vi "Trans-FPGA.vi"() -> ()   [LabVIEW 2016]
uses:
  <vilib>/LabVIEW Targets/FPGA/cRIO/shared/nicrio_ModuleControls/nicrio_cRIO-9871_BaudRateEnum.ctl
  <vilib>/LabVIEW Targets/FPGA/cRIO/shared/nicrio_ModuleControls/nicrio_cRIO-9871_DataBitsEnum.ctl
  <vilib>/LabVIEW Targets/FPGA/cRIO/shared/nicrio_ModuleControls/nicrio_cRIO-9871_ParityEnum.ctl
  <vilib>/LabVIEW Targets/FPGA/cRIO/shared/nicrio_ModuleControls/nicrio_cRIO-9871_StopBitsEnum.ctl
  <vilib>/Platform/TimedLoop/XDataNode/timing_clust.ctl
  <vilib>/Platform/TimedLoop/XDataNode/nitl_modes.ctl
  <vilib>/Platform/TimedLoop/XDataNode/wakeup.ctl
  <vilib>/rvi/FXPMathLib/basic elements/FxpIntAccumulator/subVIs/nifxpmath_IntAccumulator_SimConfig.ctl
  <vilib>/rvi/Emulation/niFpgaGetClockAttributes.vi
  <vilib>/rvi/Emulation/niFpgaSctlEmulationGetInTimedLoop.vi
  <vilib>/rvi/Emulation/niFpgaEmulationReportErrorSimple.vi
  <vilib>/rvi/eio/common/nirviEmuTemplateMethod_errors.vi
  <vilib>/rvi/Emulation/niFpgaCriticalErrorInLSC.vi
  <vilib>/rvi/Analysis/common/codeGenErrors/XNode/niFpgaXNodeCodeGenErrorHandle.vi
  <vilib>/rvi/FXPMathLib/basic elements/FxpIntAccumulator/simVIs/DllFxpIntAccumulator_sub.vi
  <vilib>/rvi/eio/common/nirviEmuTemplatePropertySet_noerrors.vi
  <vilib>/eio/EIONode/EIONode.xnode
  <vilib>/eio/EIOMethodNode/EIOMethodNode.xnode
  <vilib>/rvi/Analysis/measure/dc-rms/XNode/niFpgaDC-RMS.xnode
  <vilib>/Platform/TimedLoop/XDataNode/XDataNode.xnode
  <vilib>/rvi/FXPMathLib/basic elements/FxpIntAccumulator/XNode/nifxpmath_IntAccumulator.xnode
  <vilib>/rvi/FXPMathLib/FxpMul/XNode/nifxpmath_Multiplier.xnode
  <vilib>/eio/EIOPropertyNode/EIOPropertyNode.xnode
  <vilib>/Platform/TimedLoop/XDataNode/XDNodeRunTimeDep.lvlib
  <vilib>/rvi/FXPMathLib/sim/FxpSim.dll
  <vilib>/rvi/eio/common/nirviEmuTemplatePropertyGet_errors.vi
  <vilib>/rvi/eio/common/nirviEmuTemplatePropertyGet_noerrors.vi
  <vilib>/rvi/eio/common/nirviEmuTemplatePropertySet_errors.vi
panel:
  in  "RT error":bool
  in  "switch mag ps set":u8[](array[numeric])=[0, 0, 0, 0, 0, 0, 0, 0, 0, 0]
  out "Switch mag data":u8
  out "Timed Out 2":bool
  out "switch mag field":u8[](array[numeric])
  out "error out 2":errorcluster
  in  "trans ExB mag ps set":u8[](array[numeric])=[0, 0, 0, 0, 0, 0, 0, 0, 0, 0]
  in  "analyzer mag ps set":u8[](array[numeric])=[0, 0, 0, 0, 0, 0, 0, 0, 0, 0]
  out "analyzer mag data":u8
  out "Timed Out":bool
  out "analyzer mag field":u8[](array[numeric])
  out "error out":errorcluster
  out "Ion gauge 4":u8[](array[numeric])
  out "Convectron 4":u8[](array[numeric])
  out "Convectron 3":u8[](array[numeric])
  out "Ion gauge 3":u8[](array[numeric])
  out "Ion gauge 2":u8[](array[numeric])
  out "Convectron 2":u8[](array[numeric])
  out "Convectron 1":u8[](array[numeric])
  out "Ion gauge 1":u8[](array[numeric])
  in  "Analog Output":fxp<+/-,26,5>[](array[numeric])=[0.0, 0.0, 0.0, 0.0, 0.0, 0.0, 0.0, 0.0] format="%.23g"
  out "Analog input":fxp<+/-,26,5>[](array[numeric]) format="%.23g"
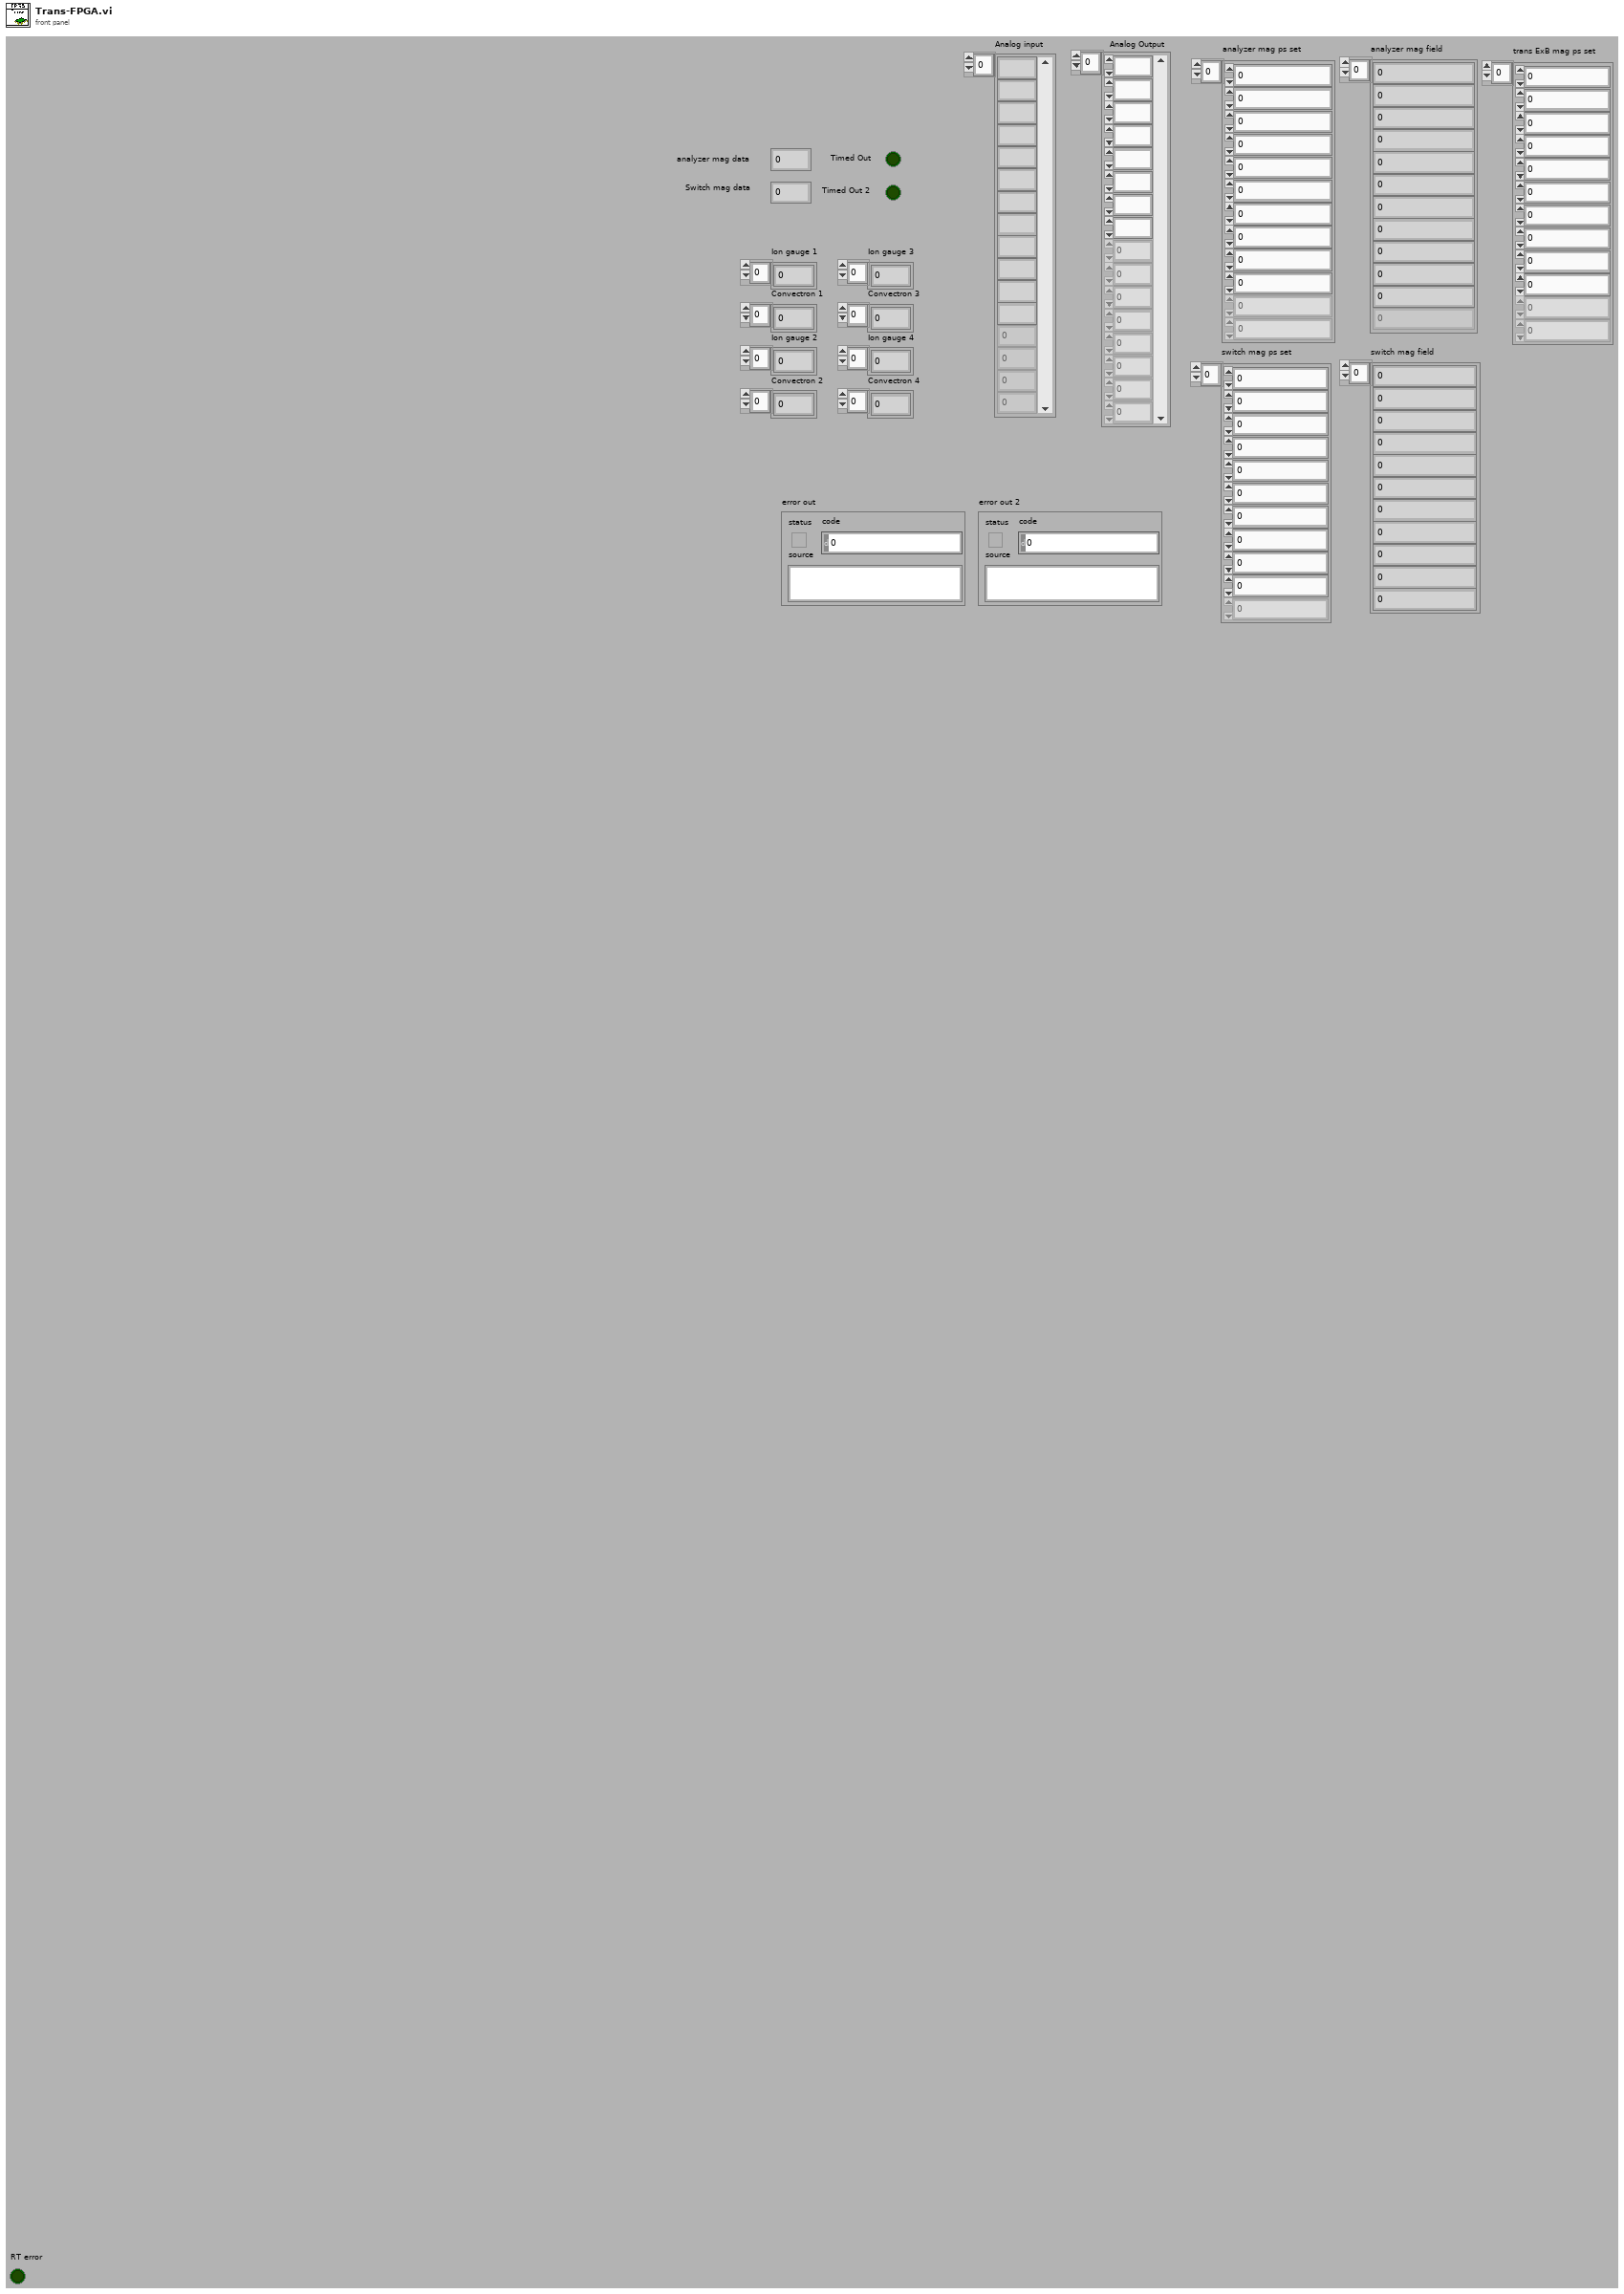
[diagram p1: front panel]
types:
  T1 = typedef "nicrio_cRIO-9871_ParityEnum.ctl" = enum8{"None", "Odd", "Even", "Mark", "Space"}
  T2 = typedef "nicrio_cRIO-9871_StopBitsEnum.ctl" = enum8{"1", "1.5", "2"}
  T3 = typedef "nicrio_cRIO-9871_BaudRateEnum.ctl" = enum16{"75 bps", "110 bps", "134 bps", "150 bps", "300 bps", "600 bps", "1200 bps", "1800 bps", "2400 bps", "4800 bps", "7200 bps", "9600 bps", "14.4 kbps", "19.2 kbps", "28.8 kbps", "38.4 kbps", "57.6 kbps", "115.2 kbps", "230.4 kbps", "460.8 kbps", "921.6 kbps"}
  T4 = typedef "nicrio_cRIO-9871_DataBitsEnum.ctl" = enum8{"5", "6", "7", "8"}
  T5 = typedef "XDNodeRunTimeDep.lvlib/timing_clust.ctl" = cluster{"Expected End [f-1]":u64, "Actual End [f-1]":u64, "Finished Late? [f-1]":bool, "Expected End [i-1]":u64, "Actual End [i-1]":u64, "Finished Late? [i-1]":bool, "Expected Start [i]":u64, "Actual Start [i]":u64, "Expected Start [f]":u64, "Actual Start [f]":u64, "Source Name":string, "Structure Name":string, "Period":i64, "Deadline":i64, "Offset":i64, "Start":i64, "Priority":i32, "Timeout":i32, "Mode":T6, "Wakeup Reason":T7, "Error":errorcluster, "Source Type":string, "Secondary Source Type":string, "Global End Time":u64, "Global Start Time":u64, "Frame Duration":u64, "Iteration Duration":u64, "Assigned CPU":i32, "I/O Scan Engine Mode":u32}
  T6 = typedef "XDNodeRunTimeDep.lvlib/nitl_modes.ctl" = enum32{"No Change", "Process missed periods, maintain original phase", "Discard missed periods, maintain original phase", "Process missed periods, ignore original phase", "Discard missed periods, ignore original phase"}
  T7 = typedef "XDNodeRunTimeDep.lvlib/wakeup.ctl" = enum32{"Normal", "Aborted", "Asynchronous wakeup", "Timing source error", "Timed loop error", "Timeout"}
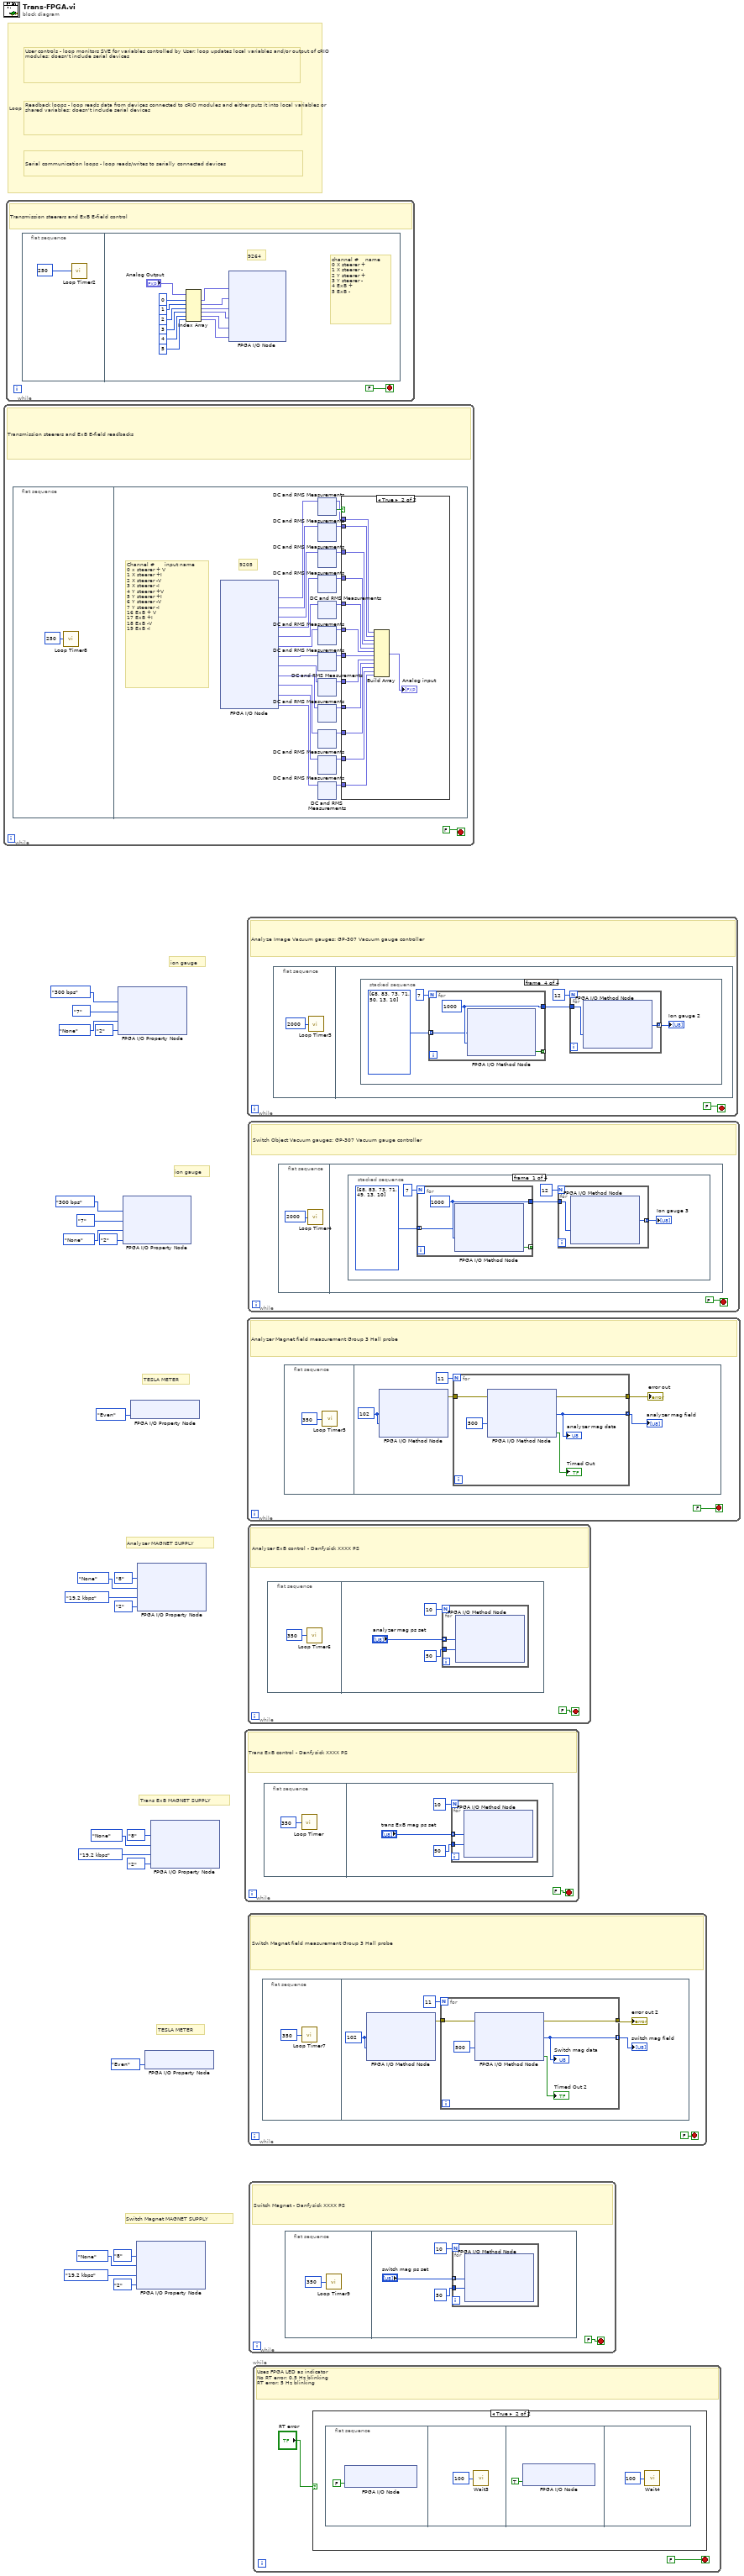
[diagram p0: block diagram]
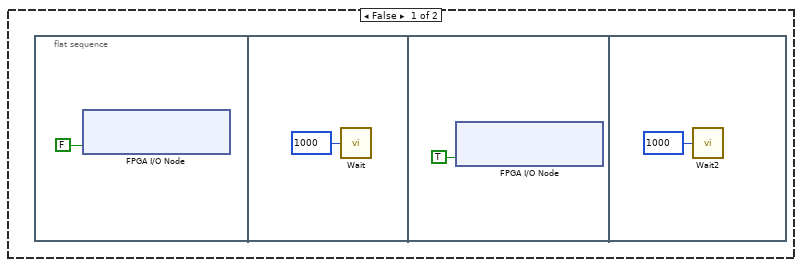
[diagram p2: hidden frame]
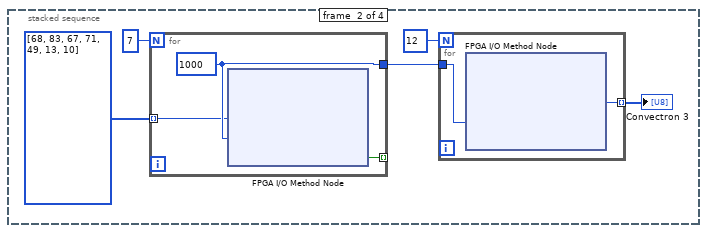
[diagram p4: hidden frame]
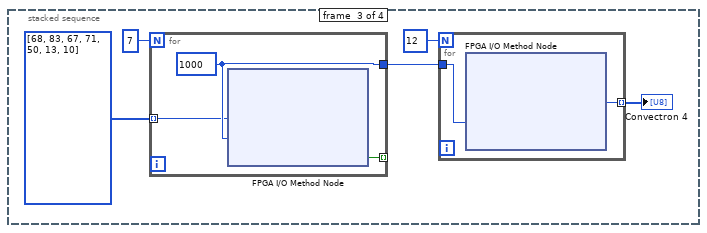
[diagram p5: hidden frame]
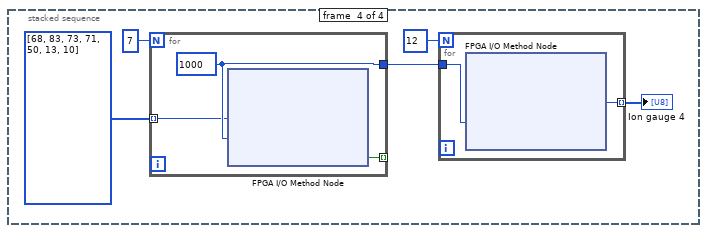
[diagram p6: hidden frame]
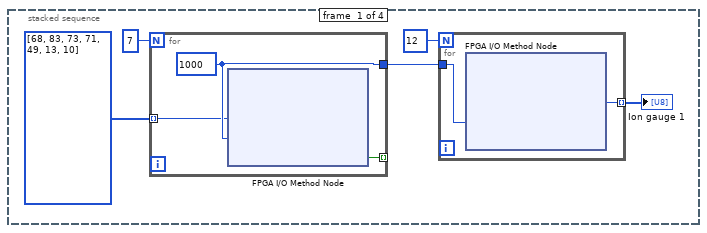
[diagram p7: hidden frame]
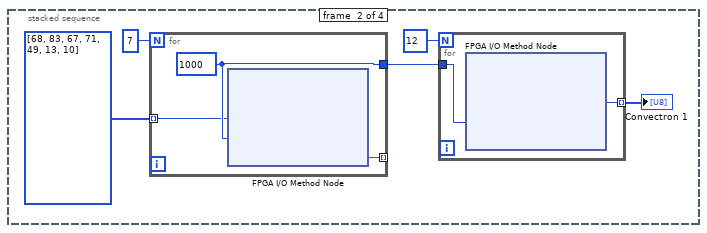
[diagram p8: hidden frame]
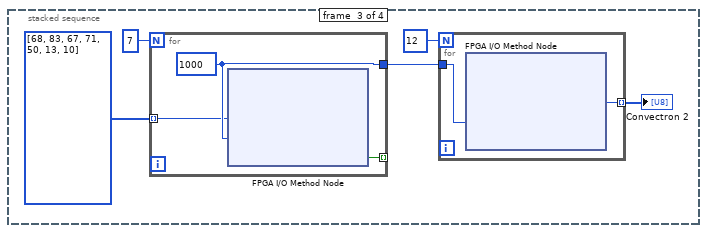
[diagram p9: hidden frame]
diagram:
  # "Serial communication loops - loop reads/writes to serially connected devices"
  # "Readback loops - loop reads data from devices connected to cRIO modules and either puts it into local variables or shared variables; doesn't include serial devices"
  # "User controls - loop monitors SVE for variables controlled by User; loop updates local variables and/or output of cRIO modules; doesn't include serial devices"
  # "Loop legend - loops are color coded by responsibility"
  # "TESLA METER"
  # "Switch Magnet MAGNET SUPPLY"
  # "Trans ExB MAGNET SUPPLY"
  # "ion gauge"
  # "Analyzer MAGNET SUPPLY"
  # "TESLA METER"
  # "ion gauge"
  n1 = while {
    stop <- FALSE stop-if-true
    # "Transmission steerers and ExB E-field readbacks"
    n2 = flat-sequence {
      frame #0 {
        n3 = call "Loop Timer8"("Count(Ticks)"=u32 250) -> ()  [unwired: 1 out]
      }
      frame #1 {
        # "Channel #      input name\n0 x steerer + V\n1 X steerer +I\n2 X steerer -V\n3 X steerer -I\n4 Y steerer +V\n5 Y steerer +I\n6 Y steerer -V\n7 Y steerer -I\n16 ExB + V\n17 ExB +I\n18 ExB -V\n19 ExB -I"
        # "9205"
        n4 = xnode "FPGA I/O Node"() -> ("Mod2/AI0"=w48:fxp<+/-,26,5>, "Mod2/AI1"=w46:fxp<+/-,26,5>, "Mod2/AI2"=w44:fxp<+/-,26,5>, "Mod2/AI3"=w42:fxp<+/-,26,5>, "Mod2/AI4"=w40:fxp<+/-,26,5>, "Mod2/AI5"=w38:fxp<+/-,26,5>, "Mod2/AI6"=w36:fxp<+/-,26,5>, "Mod2/AI7"=w34:fxp<+/-,26,5>, "Mod2/AI16"=w32:fxp<+/-,26,5>, "Mod2/AI17"=w30:fxp<+/-,26,5>, "Mod2/AI18"=w28:fxp<+/-,26,5>, "Mod2/AI19"=w26:fxp<+/-,26,5>)  [unwired: 12 in, 12 out]
        n5 = xnode "DC and RMS Measurements"("input data"=w48) -> ("DC"=w47:fxp<+/-,26,5>, "output valid"=w49:bool)  [unwired: 1 in]
        n6 = xnode "DC and RMS Measurements"("input data"=w46) -> ("DC"=w45:fxp<+/-,26,5>)  [unwired: 1 in, 1 out]
        n7 = xnode "DC and RMS Measurements"("input data"=w44) -> ("DC"=w43:fxp<+/-,26,5>)  [unwired: 1 in, 1 out]
        n8 = xnode "DC and RMS Measurements"("input data"=w42) -> ("DC"=w41:fxp<+/-,26,5>)  [unwired: 1 in, 1 out]
        n9 = xnode "DC and RMS Measurements"("input data"=w40) -> ("DC"=w39:fxp<+/-,26,5>)  [unwired: 1 in, 1 out]
        n10 = xnode "DC and RMS Measurements"("input data"=w38) -> ("DC"=w37:fxp<+/-,26,5>)  [unwired: 1 in, 1 out]
        n11 = xnode "DC and RMS Measurements"("input data"=w36) -> ("DC"=w35:fxp<+/-,26,5>)  [unwired: 1 in, 1 out]
        n12 = xnode "DC and RMS Measurements"("input data"=w34) -> ("DC"=w33:fxp<+/-,26,5>)  [unwired: 1 in, 1 out]
        n13 = xnode "DC and RMS Measurements"("input data"=w32) -> ("DC"=w31:fxp<+/-,26,5>)  [unwired: 1 in, 1 out]
        n14 = xnode "DC and RMS Measurements"("input data"=w30) -> ("DC"=w29:fxp<+/-,26,5>)  [unwired: 1 in, 1 out]
        n15 = xnode "DC and RMS Measurements"("input data"=w28) -> ("DC"=w27:fxp<+/-,26,5>)  [unwired: 1 in, 1 out]
        n16 = xnode "DC and RMS Measurements"("input data"=w26) -> ("DC"=w25:fxp<+/-,26,5>)  [unwired: 1 in, 1 out]
        n17 = case shown="True" w49 {
          tunnel: w47 -> [_ w62]
          tunnel: w45 -> [_ w61]
          tunnel: w43 -> [_ w60]
          tunnel: w41 -> [_ w59]
          tunnel: w39 -> [_ w58]
          tunnel: w37 -> [_ w57]
          tunnel: w35 -> [_ w56]
          tunnel: w33 -> [_ w55]
          tunnel: w31 -> [_ w54]
          tunnel: w29 -> [_ w53]
          tunnel: w27 -> [_ w52]
          tunnel: w25 -> [_ w51]
          frame False {
          }
          frame True {
            n18 = Build Array(w62, w61, w60, w59, w58, w57, w56, w55, w54, w53, w52, w51) -> (→"Analog input":fxp<+/-,26,5>[])
          }
        }
      }
    }
  }
  n19 = while {
    stop <- FALSE stop-if-true
    # "Transmission steerers and ExB E-field control"
    n20 = flat-sequence {
      frame #0 {
        n21 = call "Loop Timer2"("Count(uSec)"=u32 250 ("Count(Ticks)")) -> ()  [unwired: 1 out]
      }
      frame #1 {
        # "channel #    name\n0 X steerer +\n1 X steerer -\n2 Y steerer +\n3 Y steerer -\n4 ExB +\n5 ExB -"
        # "9264"
        n22 = Index Array(array="Analog Output", index #1=0 ("index"), index #2=1 ("index"), index #3=2 ("index"), index #4=3 ("index"), index #5=4 ("index"), index #6=5 ("index")) -> (element #1=w1032:fxp<+/-,26,5>, element #2=w1031:fxp<+/-,26,5>, element #3=w1030:fxp<+/-,26,5>, element #4=w1025:fxp<+/-,26,5>, element #5=w1027:fxp<+/-,26,5>, element #6=w1026:fxp<+/-,26,5>)
        n23 = xnode "FPGA I/O Node"("Mod1/AO0"=w1032, "Mod1/AO1"=w1031, "Mod1/AO2"=w1030, "Mod1/AO3"=w1025, "Mod1/AO4"=w1027, "Mod1/AO5"=w1026) -> ()  [unwired: 6 in, 6 out]
      }
    }
  }
  n24 = xnode "FPGA I/O Property Node"("Baud Rate"=nicrio_cRIO-9871_BaudRateEnum."300 bps", "Data Bits"=nicrio_cRIO-9871_DataBitsEnum."7", "Parity"=nicrio_cRIO-9871_ParityEnum."None", "Stop Bits"=nicrio_cRIO-9871_StopBitsEnum."2") -> ()  [unwired: 1 in, 1 out]
  n25 = xnode "FPGA I/O Property Node"("Baud Rate"=nicrio_cRIO-9871_BaudRateEnum."300 bps", "Data Bits"=nicrio_cRIO-9871_DataBitsEnum."7", "Parity"=nicrio_cRIO-9871_ParityEnum."None", "Stop Bits"=nicrio_cRIO-9871_StopBitsEnum."2") -> ()  [unwired: 1 in, 1 out]
  n26 = xnode "FPGA I/O Property Node"("Parity"=nicrio_cRIO-9871_ParityEnum."Even") -> ()  [unwired: 1 in, 1 out]
  n27 = xnode "FPGA I/O Property Node"("Data Bits"=nicrio_cRIO-9871_DataBitsEnum."8", "Parity"=nicrio_cRIO-9871_ParityEnum."None", "Baud Rate"=nicrio_cRIO-9871_BaudRateEnum."19.2 kbps", "Stop Bits"=nicrio_cRIO-9871_StopBitsEnum."2") -> ()  [unwired: 1 in, 1 out]
  n28 = xnode "FPGA I/O Property Node"("Data Bits"=nicrio_cRIO-9871_DataBitsEnum."8", "Parity"=nicrio_cRIO-9871_ParityEnum."None", "Baud Rate"=nicrio_cRIO-9871_BaudRateEnum."19.2 kbps", "Stop Bits"=nicrio_cRIO-9871_StopBitsEnum."2") -> ()  [unwired: 1 in, 1 out]
  n29 = xnode "FPGA I/O Property Node"("Parity"=nicrio_cRIO-9871_ParityEnum."Even") -> ()  [unwired: 1 in, 1 out]
  n30 = xnode "FPGA I/O Property Node"("Data Bits"=nicrio_cRIO-9871_DataBitsEnum."8", "Parity"=nicrio_cRIO-9871_ParityEnum."None", "Baud Rate"=nicrio_cRIO-9871_BaudRateEnum."19.2 kbps", "Stop Bits"=nicrio_cRIO-9871_StopBitsEnum."2") -> ()  [unwired: 1 in, 1 out]
  n31 = while {
    stop <- FALSE stop-if-true
    # "Trans ExB control - Danfysick XXXX PS"
    n32 = flat-sequence {
      frame #0 {
        n33 = call "Loop Timer"("Count(mSec)"=u32 350) -> ()  [unwired: 1 out]
      }
      frame #1 {
        n34 = for {
          N: 10 -> [_]
          tunnel: 50 ("Timeout (ms)") -> [w1044]
          tunnel: "trans ExB mag ps set" -> [w1043] mode=indexing
          n35 = xnode "FPGA I/O Method Node"("Data"=w1043, "Timeout (ms)"=w1044) -> ()  [unwired: 2 in, 3 out]
        }
      }
    }
  }
  n36 = while {
    stop <- FALSE stop-if-true
    # "Analyze Image Vacuum gauges: GP-307 Vacuum gauge controller"
    n37 = flat-sequence {
      frame #0 {
        n38 = call "Loop Timer3"("Count(mSec)"=u32 2000 ("Count(Ticks)")) -> ()  [unwired: 1 out]
      }
      frame #1 {
        n39 = stacked-sequence {
          frame #0 {
            n40 = for {
              N: 7 -> [_]
              tunnel: [w1056] -> w1051
              tunnel: [w1055] -> _ mode=indexing
              tunnel: u8[] [68, 83, 73, 71, 49, 13, 10] ("unsigned byte array") -> [w1054] mode=indexing
              w1056 = 1000 ("Timeout (ms)")
              n41 = xnode "FPGA I/O Method Node"("Data"=w1054, "Timeout (ms)"=w1056) -> ("Timed Out"=w1055:bool)  [unwired: 1 in, 1 out]
            }
            n42 = for {
              N: 12 -> [_]
              tunnel: w1051 -> [w1053]
              tunnel: [w1052] -> w1047 mode=indexing
              n43 = xnode "FPGA I/O Method Node"("Timeout (ms)"=w1053) -> ("Data"=w1052:u8)  [unwired: 1 in, 2 out]
            }
            "Ion gauge 1" <- w1047
          }
          frame #1 {
            n44 = for {
              N: 7 -> [_]
              tunnel: [w1066] -> w1061
              tunnel: [w1065] -> _ mode=indexing
              tunnel: u8[] [68, 83, 67, 71, 49, 13, 10] ("unsigned byte array") -> [w1064] mode=indexing
              w1066 = 1000 ("Timeout (ms)")
              n45 = xnode "FPGA I/O Method Node"("Data"=w1064, "Timeout (ms)"=w1066) -> ("Timed Out"=w1065:bool)  [unwired: 1 in, 1 out]
            }
            n46 = for {
              N: 12 -> [_]
              tunnel: w1061 -> [w1063]
              tunnel: [w1062] -> w1057 mode=indexing
              n47 = xnode "FPGA I/O Method Node"("Timeout (ms)"=w1063) -> ("Data"=w1062:u8)  [unwired: 1 in, 2 out]
            }
            "Convectron 1" <- w1057
          }
          frame #2 {
            n48 = for {
              N: 7 -> [_]
              tunnel: [w1076] -> w1071
              tunnel: [w1075] -> _ mode=indexing
              tunnel: u8[] [68, 83, 67, 71, 50, 13, 10] ("unsigned byte array") -> [w1074] mode=indexing
              w1076 = 1000 ("Timeout (ms)")
              n49 = xnode "FPGA I/O Method Node"("Data"=w1074, "Timeout (ms)"=w1076) -> ("Timed Out"=w1075:bool)  [unwired: 1 in, 1 out]
            }
            n50 = for {
              N: 12 -> [_]
              tunnel: w1071 -> [w1073]
              tunnel: [w1072] -> w1067 mode=indexing
              n51 = xnode "FPGA I/O Method Node"("Timeout (ms)"=w1073) -> ("Data"=w1072:u8)  [unwired: 1 in, 2 out]
            }
            "Convectron 2" <- w1067
          }
          frame #3 {
            n52 = for {
              N: 7 -> [_]
              tunnel: [w1086] -> w1081
              tunnel: [w1085] -> _ mode=indexing
              tunnel: u8[] [68, 83, 73, 71, 50, 13, 10] ("unsigned byte array") -> [w1084] mode=indexing
              w1086 = 1000 ("Timeout (ms)")
              n53 = xnode "FPGA I/O Method Node"("Data"=w1084, "Timeout (ms)"=w1086) -> ("Timed Out"=w1085:bool)  [unwired: 1 in, 1 out]
            }
            n54 = for {
              N: 12 -> [_]
              tunnel: w1081 -> [w1083]
              tunnel: [w1082] -> w1077 mode=indexing
              n55 = xnode "FPGA I/O Method Node"("Timeout (ms)"=w1083) -> ("Data"=w1082:u8)  [unwired: 1 in, 2 out]
            }
            "Ion gauge 2" <- w1077
          }
        }
      }
    }
  }
  n56 = while {
    stop <- FALSE stop-if-true
    # "Analyzer Magnet field measurement Group 3 Hall probe"
    n57 = flat-sequence {
      frame #0 {
        n58 = call "Loop Timer5"("Count(mSec)"=u32 350) -> ()  [unwired: 1 out]
      }
      frame #1 {
        w1092 = u8 102 ("Data")
        n59 = xnode "FPGA I/O Method Node"("Data"=w1092, "Timeout (ms)"=w1092) -> ("error out"=w1091:errorcluster)  [unwired: 2 in, 2 out]
        n60 = for {
          N: 11 ("Numeric 3") -> [_]
          tunnel: [w1096] -> w1089 mode=indexing
          tunnel: w1091 -> [w1095]
          tunnel: [w1094] -> w1090
          n61 = xnode "FPGA I/O Method Node"("error in"=w1095, "Timeout (ms)"=500) -> ("error out"=w1094:errorcluster, "Data"=w1096:u8, "Timed Out"=→"Timed Out":bool)  [unwired: 1 in, 1 out]
          "analyzer mag data" <- w1096
        }
        "analyzer mag field" <- w1089
        "error out" <- w1090
      }
    }
  }
  n62 = while {
    stop <- FALSE stop-if-true
    # "Analyzer ExB control - Danfysick XXXX PS"
    n63 = flat-sequence {
      frame #0 {
        n64 = call "Loop Timer6"("Count(mSec)"=u32 350) -> ()  [unwired: 1 out]
      }
      frame #1 {
        n65 = for {
          N: 10 -> [_]
          tunnel: 50 ("Timeout (ms)") -> [w1105]
          tunnel: "analyzer mag ps set" -> [w1104] mode=indexing
          n66 = xnode "FPGA I/O Method Node"("Data"=w1104, "Timeout (ms)"=w1105) -> ()  [unwired: 2 in, 3 out]
        }
      }
    }
  }
  n67 = while {
    stop <- FALSE stop-if-true
    # "Switch Magnet field measurement Group 3 Hall probe"
    n68 = flat-sequence {
      frame #0 {
        n69 = call "Loop Timer7"("Count(mSec)"=u32 350) -> ()  [unwired: 1 out]
      }
      frame #1 {
        w1111 = u8 102 ("Data")
        n70 = xnode "FPGA I/O Method Node"("Data"=w1111, "Timeout (ms)"=w1111) -> ("error out"=w1110:errorcluster)  [unwired: 2 in, 2 out]
        n71 = for {
          N: 11 ("Numeric 3") -> [_]
          tunnel: [w1115] -> w1108 mode=indexing
          tunnel: w1110 -> [w1114]
          tunnel: [w1113] -> w1109
          n72 = xnode "FPGA I/O Method Node"("error in"=w1114, "Timeout (ms)"=500) -> ("error out"=w1113:errorcluster, "Data"=w1115:u8, "Timed Out"=→"Timed Out 2":bool)  [unwired: 1 in, 1 out]
          "Switch mag data" <- w1115
        }
        "switch mag field" <- w1108
        "error out 2" <- w1109
      }
    }
  }
  n73 = while {
    stop <- FALSE stop-if-true
    # "Switch Object Vacuum gauges: GP-307 Vacuum gauge controller"
    n74 = flat-sequence {
      frame #0 {
        n75 = call "Loop Timer4"("Count(mSec)"=u32 2000 ("Count(Ticks)")) -> ()  [unwired: 1 out]
      }
      frame #1 {
        n76 = stacked-sequence {
          frame #0 {
            n77 = for {
              N: 7 -> [_]
              tunnel: [w1129] -> w1124
              tunnel: [w1128] -> _ mode=indexing
              tunnel: u8[] [68, 83, 73, 71, 49, 13, 10] ("unsigned byte array") -> [w1127] mode=indexing
              w1129 = 1000 ("Timeout (ms)")
              n78 = xnode "FPGA I/O Method Node"("Data"=w1127, "Timeout (ms)"=w1129) -> ("Timed Out"=w1128:bool)  [unwired: 1 in, 1 out]
            }
            n79 = for {
              N: 12 -> [_]
              tunnel: w1124 -> [w1126]
              tunnel: [w1125] -> w1120 mode=indexing
              n80 = xnode "FPGA I/O Method Node"("Timeout (ms)"=w1126) -> ("Data"=w1125:u8)  [unwired: 1 in, 2 out]
            }
            "Ion gauge 3" <- w1120
          }
          frame #1 {
            n81 = for {
              N: 7 -> [_]
              tunnel: [w1139] -> w1134
              tunnel: [w1138] -> _ mode=indexing
              tunnel: u8[] [68, 83, 67, 71, 49, 13, 10] ("unsigned byte array") -> [w1137] mode=indexing
              w1139 = 1000 ("Timeout (ms)")
              n82 = xnode "FPGA I/O Method Node"("Data"=w1137, "Timeout (ms)"=w1139) -> ("Timed Out"=w1138:bool)  [unwired: 1 in, 1 out]
            }
            n83 = for {
              N: 12 -> [_]
              tunnel: w1134 -> [w1136]
              tunnel: [w1135] -> w1130 mode=indexing
              n84 = xnode "FPGA I/O Method Node"("Timeout (ms)"=w1136) -> ("Data"=w1135:u8)  [unwired: 1 in, 2 out]
            }
            "Convectron 3" <- w1130
          }
          frame #2 {
            n85 = for {
              N: 7 -> [_]
              tunnel: [w1149] -> w1144
              tunnel: [w1148] -> _ mode=indexing
              tunnel: u8[] [68, 83, 67, 71, 50, 13, 10] ("unsigned byte array") -> [w1147] mode=indexing
              w1149 = 1000 ("Timeout (ms)")
              n86 = xnode "FPGA I/O Method Node"("Data"=w1147, "Timeout (ms)"=w1149) -> ("Timed Out"=w1148:bool)  [unwired: 1 in, 1 out]
            }
            n87 = for {
              N: 12 -> [_]
              tunnel: w1144 -> [w1146]
              tunnel: [w1145] -> w1140 mode=indexing
              n88 = xnode "FPGA I/O Method Node"("Timeout (ms)"=w1146) -> ("Data"=w1145:u8)  [unwired: 1 in, 2 out]
            }
            "Convectron 4" <- w1140
          }
          frame #3 {
            n89 = for {
              N: 7 -> [_]
              tunnel: [w1159] -> w1154
              tunnel: [w1158] -> _ mode=indexing
              tunnel: u8[] [68, 83, 73, 71, 50, 13, 10] ("unsigned byte array") -> [w1157] mode=indexing
              w1159 = 1000 ("Timeout (ms)")
              n90 = xnode "FPGA I/O Method Node"("Data"=w1157, "Timeout (ms)"=w1159) -> ("Timed Out"=w1158:bool)  [unwired: 1 in, 1 out]
            }
            n91 = for {
              N: 12 -> [_]
              tunnel: w1154 -> [w1156]
              tunnel: [w1155] -> w1150 mode=indexing
              n92 = xnode "FPGA I/O Method Node"("Timeout (ms)"=w1156) -> ("Data"=w1155:u8)  [unwired: 1 in, 2 out]
            }
            "Ion gauge 4" <- w1150
          }
        }
      }
    }
  }
  n93 = while {
    stop <- FALSE stop-if-true
    # "Switch Magnet - Danfysick XXXX PS"
    n94 = flat-sequence {
      frame #0 {
        n95 = call "Loop Timer9"("Count(mSec)"=u32 350) -> ()  [unwired: 1 out]
      }
      frame #1 {
        n96 = for {
          N: 10 -> [_]
          tunnel: 50 ("Timeout (ms)") -> [w1166]
          tunnel: "switch mag ps set" -> [w1165] mode=indexing
          n97 = xnode "FPGA I/O Method Node"("Data"=w1165, "Timeout (ms)"=w1166) -> ()  [unwired: 2 in, 3 out]
        }
      }
    }
  }
  n98 = while {
    stop <- FALSE stop-if-true
    # "Uses FPGA LED as indicator\nNo RT error: 0.5 Hz blinking\nRT error: 5 Hz blinking"
    n99 = case shown="True" "RT error" {
      frame False {
        n100 = flat-sequence {
          frame #0 {
            n101 = xnode "FPGA I/O Node"("USER FPGA LED"=FALSE ("FPGA LED")) -> ()  [unwired: 1 in, 1 out]
          }
          frame #1 {
            n102 = call "Wait"("Count(mSec)"=u16 1000) -> ()  [unwired: 1 out]
          }
          frame #2 {
            n103 = xnode "FPGA I/O Node"("USER FPGA LED"=TRUE ("FPGA LED")) -> ()  [unwired: 1 in, 1 out]
          }
          frame #3 {
            n104 = call "Wait2"("Count(mSec)"=u16 1000) -> ()  [unwired: 1 out]
          }
        }
      }
      frame True {
        n105 = flat-sequence {
          frame #0 {
            n106 = xnode "FPGA I/O Node"("USER FPGA LED"=FALSE ("FPGA LED")) -> ()  [unwired: 1 in, 1 out]
          }
          frame #1 {
            n107 = call "Wait3"("Count(mSec)"=u16 100) -> ()  [unwired: 1 out]
          }
          frame #2 {
            n108 = xnode "FPGA I/O Node"("USER FPGA LED"=TRUE ("FPGA LED")) -> ()  [unwired: 1 in, 1 out]
          }
          frame #3 {
            n109 = call "Wait4"("Count(mSec)"=u16 100) -> ()  [unwired: 1 out]
          }
        }
      }
    }
  }
